vi "Query All Plugins.vi"(6 "timeout (ms)":i32=5000, 8 "error in":errorcluster, 11 "gRPC ID in":T12) -> (0 "error out":errorcluster, 2 "plugin_info":T1[](array[typedef]) {"Node Status"."Monitor Doubles"."4" format="%#_9g"; "Node Status"."Monitor Doubles"."3" format="%#_9g"; "Node Status"."Monitor Doubles"."2" format="%#_9g"; "Node Status"."Monitor Doubles"."1" format="%#_9g"; "Node Status"."Timing Statistics (us)"."Period"."Avg" format="%_6g"}, 3 "gRPC ID out":T12)   [LabVIEW 2021, in "CIFManagerClientWrapper.lvlib"]
uses:
  CIFManagerClientWrapper.lvlib
  <vilib>/gRPC/LabVIEW gRPC Library/Shared/grpcId.ctl
  CIFCore/Common/Typedef/PluginInfo.ctl
  CIFCore/Common/Typedef/Version Simple.ctl
  CIFCore/Common/Typedef/gRPC Reported Plugin Status.ctl
  CIFCore/Common/Typedef/Plugin State.ctl
  CIFCore/Common/Typedef/Timing Statistics.ctl
  CIFCore/Common/Typedef/Timing Stats Base.ctl
  CIFCore/Common/Typedef/FIFO Statistics.ctl
  CIFCore/Common/Typedef/Simple Error.ctl
  CIFCore/Common/Typedef/Monitor Doubles.ctl
  CIFCore/Common/Typedef/Monitor U64.ctl
  CIFCore/Common/Typedef/Monitor I64.ctl
  CIF_Manager_client/RPC Messages/cif_manager_QueryPluginInfoRequest.ctl
  CIF_Manager_client/CIF_Manager_client.lvlib
  CIFCore/Grpc/CIFCoreWrapper/CIFCoreWrapper.lvlib
  CIFCore/Common/CIFCoreCommon.lvlib
  <vilib>/gRPC/LabVIEW gRPC Library/grpc-lvsupport-release.lvlib
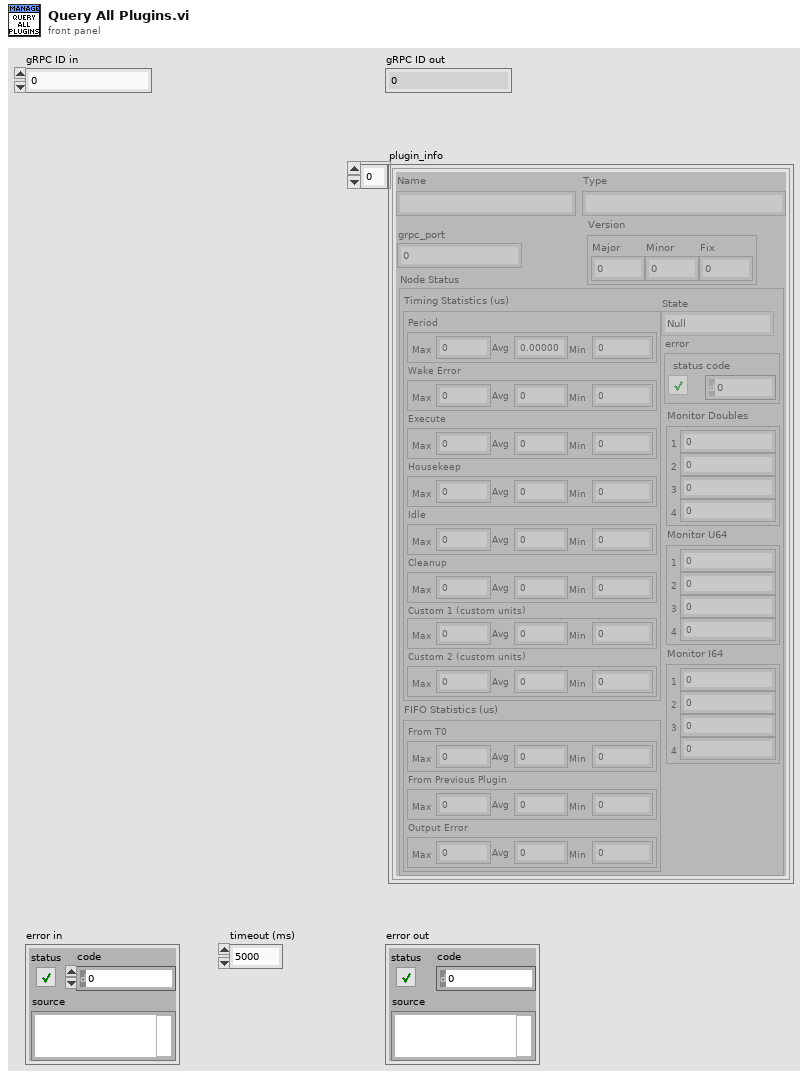
[diagram p1: front panel]
types:
  T1 = typedef "CIFCoreCommon.lvlib/PluginInfo.ctl" = cluster{"Name":string, "Type":string, "grpc_port":i32, "Version":T2, "Node Status":T3}
  T2 = typedef "CIFCoreCommon.lvlib/Version Simple.ctl" = cluster{"Major":i32, "Minor":i32, "Fix":i32}
  T3 = typedef "CIFCoreCommon.lvlib/gRPC Reported Plugin Status.ctl" = cluster{"State":T4, "Timing Statistics (us)":T5, "FIFO Statistics (us)":T7, "error":T8, "Monitor Doubles":T9, "Monitor U64":T10, "Monitor I64":T11}
  T4 = typedef "CIFCoreCommon.lvlib/Plugin State.ctl" = enum32{"Null", "Creating", "Listening", "Running", "CleaningUp", "Destroying"}
  T5 = typedef "CIFCoreCommon.lvlib/Timing Statistics.ctl" = cluster{"Period":T6, "Wake Error":T6, "Execute":T6, "Housekeep":T6, "Idle":T6, "Cleanup":T6, "Custom 1 (custom units)":T6, "Custom 2 (custom units)":T6}
  T6 = typedef "CIFCoreCommon.lvlib/Timing Stats Base.ctl" = cluster{"Max":i64, "Avg":dbl, "Min":i64}
  T7 = typedef "CIFCoreCommon.lvlib/FIFO Statistics.ctl" = cluster{"From T0":T6, "From Previous Plugin":T6, "Output Error":T6}
  T8 = typedef "CIFCoreCommon.lvlib/Simple Error.ctl" = cluster{"status":bool, "code":i32}
  T9 = typedef "CIFCoreCommon.lvlib/Monitor Doubles.ctl" = cluster{"1":dbl, "2":dbl, "3":dbl, "4":dbl}
  T10 = typedef "CIFCoreCommon.lvlib/Monitor U64.ctl" = cluster{"1":u64, "2":u64, "3":u64, "4":u64}
  T11 = typedef "CIFCoreCommon.lvlib/Monitor I64.ctl" = cluster{"1":i64, "2":i64, "3":i64, "4":i64}
  T12 = typedef "grpc-lvsupport-release.lvlib/grpcId.ctl" = u64
  T13 = typedef "CIF_Manager_client.lvlib/cif_manager_QueryPluginInfoRequest.ctl" = cluster{"void":string}
  T14 = typedef "CIF_Manager_client.lvlib/cif_manager_QueryPluginInfoResponse.ctl" = cluster{"plugin_info_array":T15}
  T15 = typedef "CIF_Manager_client.lvlib/cif_manager_PluginInfoArray.ctl" = cluster{"plugin_info":T16[]}
  T16 = typedef "CIF_Manager_client.lvlib/cif_manager_PluginInfo.ctl" = cluster{"plugin_name":string, "plugin_type":string, "grpc_port":i32, "plugin_version":T17, "status":T18, "loader_info":T27}
  T17 = typedef "CIF_Manager_client.lvlib/cif_common_ShortVersion.ctl" = cluster{"major":u32, "minor":u32, "fix":u32}
  T18 = typedef "CIF_Manager_client.lvlib/cif_management_common_PluginStatusData.ctl" = cluster{"state":T19, "timing_statistics":T20, "fifo_statistics":T22, "error":T23, "monitor_doubles":T24, "monitor_u64s":T25, "monitor_i64s":T26}
  T19 = typedef "CIF_Manager_client.lvlib/cif_management_common_PluginStatusData_PluginState.ctl" = enum32{"PLUGINSTATE_UNKNOWN", "PLUGINSTATE_CREATING", "PLUGINSTATE_LISTENING", "PLUGINSTATE_RUNNING", "PLUGINSTATE_CLEANINGUP", "PLUGINSTATE_DESTROYING"}
  T20 = typedef "CIF_Manager_client.lvlib/cif_management_common_TimingStatistics.ctl" = cluster{"period":T21, "wake_error":T21, "execute":T21, "housekeep":T21, "idle":T21, "cleanup":T21, "custom_1":T21, "custom_2":T21}
  T21 = typedef "CIF_Manager_client.lvlib/cif_common_TimingStats.ctl" = cluster{"max":i64, "min":i64, "avg":dbl}
  T22 = typedef "CIF_Manager_client.lvlib/cif_management_common_FifoStatistics.ctl" = cluster{"from_t0":T21, "from_previous_plugin":T21, "output_error":T21}
  T23 = typedef "CIF_Manager_client.lvlib/cif_management_common_Error.ctl" = cluster{"status":bool, "code":i32}
  T24 = typedef "CIF_Manager_client.lvlib/cif_management_common_MonitorDoubles.ctl" = cluster{"double_1":dbl, "double_2":dbl, "double_3":dbl, "double_4":dbl}
  T25 = typedef "CIF_Manager_client.lvlib/cif_management_common_MonitorU64.ctl" = cluster{"u64_1":u64, "u64_2":u64, "u64_3":u64, "u64_4":u64}
  T26 = typedef "CIF_Manager_client.lvlib/cif_management_common_MonitorI64.ctl" = cluster{"i64_1":i64, "i64_2":i64, "i64_3":i64, "i64_4":i64}
  T27 = typedef "CIF_Manager_client.lvlib/cif_management_common_LoaderInfo.ctl" = cluster{"loader_type":T28, "loader_name":string}
  T28 = typedef "CIF_Manager_client.lvlib/cif_management_common_LoaderType.ctl" = enum32{"LOADERTYPE_UNKNOWN", "LOADERTYPE_LABVIEW"}
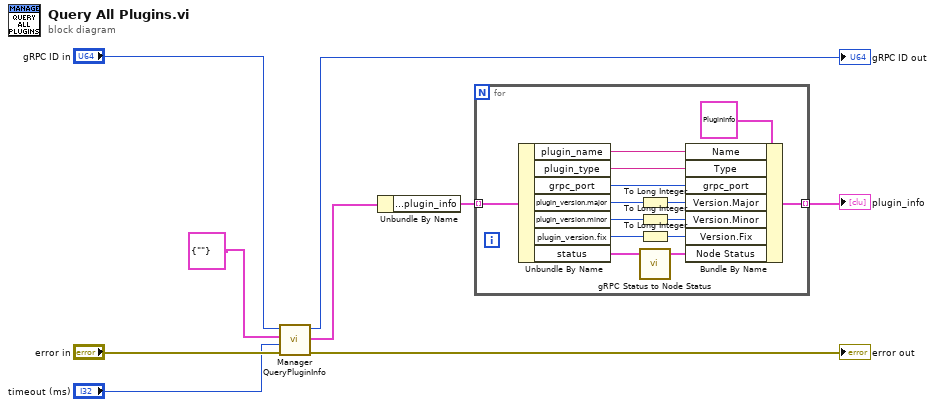
[diagram p0: block diagram]
diagram:
  n1 = call "Manager QueryPluginInfo.vi"("error in"="error in", "timeout (ms)"="timeout (ms)", "Request Data"=T13 {"void"=""}, "gRPC ID"="gRPC ID in") -> ("error out"=→"error out":errorcluster, "Response Data"=w5:T14, "gRPC ID out"=→"gRPC ID out":T12)  [unwired: 5 in]
  n2 = Unbundle By Name(w5) -> ("plugin_info_array.plugin_info"=w3:T16[])
  n3 = for {
    tunnel: w3 -> [w23] mode=indexing
    tunnel: [w13] -> w2 mode=indexing
    n4 = Unbundle By Name(w23) -> ("plugin_name"=w21:string, "plugin_type"=w14:string, "grpc_port"=w15:i32, "plugin_version.major"=w16:u32, "plugin_version.minor"=w17:u32, "plugin_version.fix"=w18:u32, "status"=w20:T18)
    n5 = To Long Integer(number=w16) -> (32bit integer=w12:i32)
    n6 = To Long Integer(number=w17) -> (32bit integer=w11:i32)
    n7 = To Long Integer(number=w18) -> (32bit integer=w10:i32)
    n8 = call "gRPC Status to Node Status.vi"("gRPC Status"=w20) -> ("Node Status"=w19:T3)  [unwired: 3 in]
    n9 = Bundle By Name(cluster=T1 {"Name"="", "Type"="", "grpc_port"=0, "Version"={"Major"=0, "Minor"=0, "Fix"=0}, "Node Status"={"State"=enum."Null", "Timing Statistics (us)"={"Period"={"Max"=0, "Avg"=0.0, "Min"=0}, "Wake Error"={"Max"=0, "Avg"=0.0, "Min"=0}, "Execute"={"Max"=0, "Avg"=0.0, "Min"=0}, "Housekeep"={"Max"=0, "Avg"=0.0, "Min"=0}, "Idle"={"Max"=0, "Avg"=0.0, "Min"=0}, "Cleanup"={"Max"=0, "Avg"=0.0, "Min"=0}, "Custom 1 (custom units)"={"Max"=0, "Avg"=0.0, "Min"=0}, "Custom 2 (custom units)"={"Max"=0, "Avg"=0.0, "Min"=0}}, "FIFO Statistics (us)"={"From T0"={"Max"=0, "Avg"=0.0, "Min"=0}, "From Previous Plugin"={"Max"=0, "Avg"=0.0, "Min"=0}, "Output Error"={"Max"=0, "Avg"=0.0, "Min"=0}}, "error"={"status"=FALSE, "code"=0}, "Monitor Doubles"={"1"=0.0, "2"=0.0, "3"=0.0, "4"=0.0}, "Monitor U64"={"1"=0, "2"=0, "3"=0, "4"=0}, "Monitor I64"={"1"=0, "2"=0, "3"=0, "4"=0}}} ("Plugin Info"), "Name"=w21, "Type"=w14, "grpc_port"=w15, "Version.Major"=w12, "Version.Minor"=w11, "Version.Fix"=w10, "Node Status"=w19) -> (w13:T1)
  }
  "plugin_info" <- w2
